vi "Up_SN.vi"(0 "Image Src":T8, 5 "ROIIn":string, 11 "error in":errorcluster) -> (4 "Image Out":T8(plugin-control), 6 "QR Code Report":T1={"Found?"=FALSE, "Data"="", "Bounding Box"=[], "Errors Corrected"=0, "Dimensions (Rows/Cols)"=0, "Version"=0, "QR Model"=0, "Stream Mode"=0, "Barcode Polarity"=-2, "Mirrored?"=FALSE, "Append Stream Position"=0, "Size of Append Stream"=0, "First EAN-128 ID"=0, "First Alternate Language ID"=0, "Append Stream ID"=0, "Minimum Edge Strength"=30, "Demodulation Mode"=-2, "Cell Sample Size"=-2, "Cell Filter Mode"=-2} {"Append Stream ID" format="%x"; "Cell Filter Mode" items=["Auto-detect"=-2, "Average"=0, "Median"=1, "Central Average"=2, "High Average"=3, "Low Average"=4, "Very High Average"=5, "Very Low Average"=6, "All Filters"=8]; "Cell Sample Size" items=["Auto-detect"=-2, "1x1"=1, "2x2"=2, "3x3"=3, "4x4"=4, "5x5"=5, "6x6"=6, "7x7"=7]; "Demodulation Mode" items=["Auto-detect"=-2, "Histogram"=0, "Local Contrast"=1, "Combination"=2, "All"=3]; "Barcode Polarity" items=["Auto-detect"=-2, "Black on White"=0, "White on Black"=1]; "Stream Mode" items=["Numeric", "AlphaNumeric", "Raw Bytes", "UCC/EAN-128 - In Tokens", "UCC/EAN-128 - In Data", "Extended Character Interpretation", "Kanji"]; "QR Model" items=["Auto-detect", "Micro", "Model 1", "Model 2"]; "Version" max=40 step=1}, 15 "error out":errorcluster)   [LabVIEW 2019]
uses:
  <vilib>/vision/Image Controls.llb/IMAQ Image.ctl
  <vilib>/vision/Instrument.llb/QR Code Report.ctl
  <vilib>/vision/Instrument.llb/QR Code Model Type.ctl
  <vilib>/vision/Instrument.llb/QR Code Stream Mode Type.ctl
  <vilib>/vision/Instrument.llb/Data Matrix Polarity.ctl
  <vilib>/vision/Instrument.llb/Demodulation Mode.ctl
  <vilib>/vision/Instrument.llb/Cell Sample Size.ctl
  <vilib>/vision/Instrument.llb/Cell Filter Mode.ctl
  <vilib>/vision/NI_Vision_Development_Module.lvlib
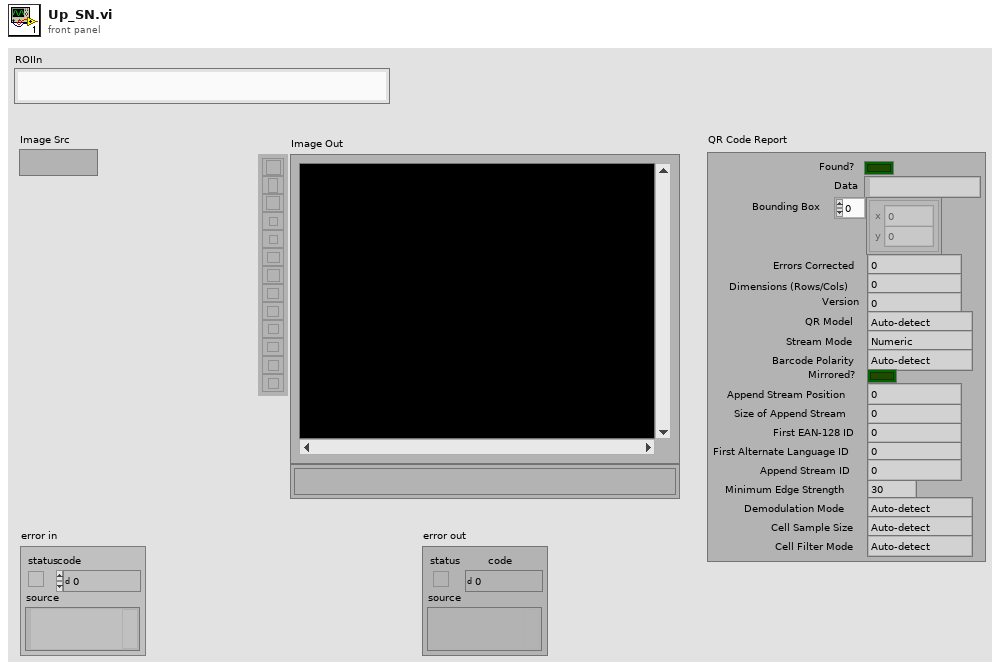
[diagram p1: front panel]
types:
  T1 = typedef "QR Code Report.ctl" = cluster{"Found?":bool, "Data":string, "Bounding Box":cluster{"x":sgl, "y":sgl}[], "Errors Corrected":u32, "Dimensions (Rows/Cols)":u32, "Version":u32, "QR Model":T2, "Stream Mode":T3, "Barcode Polarity":T4, "Mirrored?":bool, "Append Stream Position":u32, "Size of Append Stream":u32, "First EAN-128 ID":i32, "First Alternate Language ID":i32, "Append Stream ID":u32, "Minimum Edge Strength":u32, "Demodulation Mode":T5, "Cell Sample Size":T6, "Cell Filter Mode":T7}
  T2 = typedef "QR Code Model Type.ctl" = i32
  T3 = typedef "QR Code Stream Mode Type.ctl" = i32
  T4 = typedef "Data Matrix Polarity.ctl" = i32
  T5 = typedef "Demodulation Mode.ctl" = i32
  T6 = typedef "Cell Sample Size.ctl" = i32
  T7 = typedef "Cell Filter Mode.ctl" = i32
  T8 = typedef "IMAQ Image.ctl" = refnum<image>
  T9 = cluster{"Rotation Mode":enum32{"Unlimited", "0 Degrees", "90 Degrees", "180 Degrees", "270 Degrees"}, "Skip Location?":bool, "Edge Threshold":u32, "Demodulation Mode":i32, "Cell Sample Size":i32, "Cell Filter Mode":i32, "Skew Degrees Allowed":u32}[]
  T10 = typedef "Image Type" = u32
  T11 = typedef "IMAQ Rectangle" = cluster{"Left":i32, "Top":i32, "Right":i32, "Bottom":i32, "Rotation":dbl}
  T12 = cluster{"Matrix Dimensions (cells)":i32, "Barcode Polarity":i32, "Mirror Mode":i32, "QR Model":i32}
  T13 = cluster{"Rotation Mode":enum32{"Unlimited", "0 Degrees", "90 Degrees", "180 Degrees", "270 Degrees"}, "Skip Location?":bool, "Edge Threshold":u32, "Demodulation Mode":i32, "Cell Sample Size":i32, "Cell Filter Mode":i32, "Skew Degrees Allowed":u32}
  T14 = typedef "ROI Descriptor" = cluster{"Global Rectangle":i32[], "Contours":cluster{"ID":enum32{"External", "Internal"}, "Type":u32, "Coordinates":i32[]}[]}
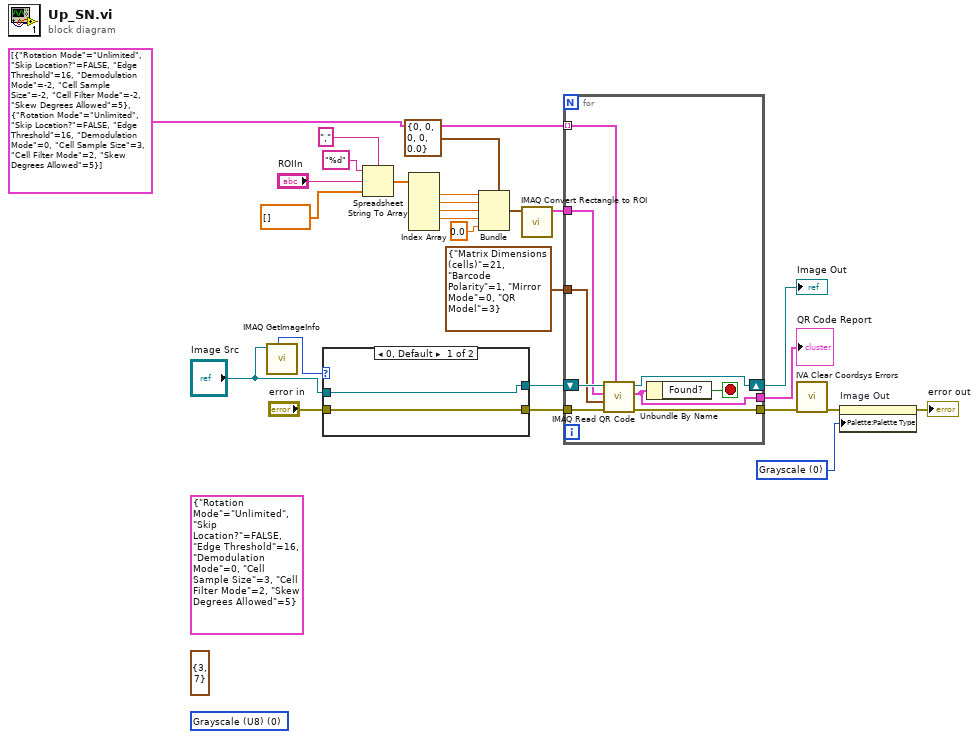
[diagram p0: block diagram]
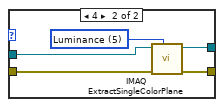
[diagram p2: hidden frame]
diagram:
  (unwired) T10 0 items=["Grayscale (U8)", "Grayscale (I16)", "Grayscale (SGL)", "Complex (CSG)", "RGB (U32)", "HSL (U32)", "RGB (U64)", "Grayscale (U16)"] ("Image Type")
  w19 = u32 0 items=["Grayscale", "Binary", "Gradient", "Rainbow", "Temperature", "User Defined", "Binary 16 Bit", "Gradient 16 Bit", "Rainbow 16 Bit", "Temperature 16 Bit", "User Defined 16 Bit"] ("Palette Type")
  (unwired) cluster{"Minimum Size":u32, "Maximum Size":u32} {"Minimum Size"=3, "Maximum Size"=7} ("QR Code Cell Size (pixels)")
  (unwired) T13 {"Rotation Mode"=enum."Unlimited", "Skip Location?"=FALSE, "Edge Threshold"=16, "Demodulation Mode"=0, "Cell Sample Size"=3, "Cell Filter Mode"=2, "Skew Degrees Allowed"=5} ("QR Search Options")
  n1 = call "IMAQ GetImageInfo"("Image"="Image Src") -> ("Image Type"=w3:T10)  [unwired: 3 in, 7 out]
  n2 = case shown="0, Default" w3 {
    tunnel: [w27 w32] -> w26
    tunnel: [w28 w31] -> w25
    tunnel: "error in" -> [w27 w30]
    tunnel: "Image Src" -> [w28 w29]
    frame 0, Default {
    }
    frame 4 {
      w33 = 5 items=["Red", "Green", "Blue", "Hue", "Saturation", "Luminance", "Value", "Intensity"] ("Color Plane")
      n3 = call "IMAQ ExtractSingleColorPlane"("Color Plane"=w33, "error in (no error)"=w30, "Image Src"=w29) -> ("error out"=w32:errorcluster, "Image Dst Out"=w31:T8)  [unwired: 1 in, 6 out]
    }
  }
  n4 = Spreadsheet String To Array(delimiter (Tab)=",", format string="%d", spreadsheet string="ROIIn", array type (2D Dbl)=dbl[] []) -> (array=w11:dbl[])
  n5 = Index Array(array=w11) -> (element #1=w10:dbl, element #2=w9:dbl, element #3=w8:dbl, element #4=w7:dbl)  [unwired: 5 in, 1 out]
  n6 = Bundle(cluster=T11 {"Left"=0, "Top"=0, "Right"=0, "Bottom"=0, "Rotation"=0.0} ("Rectangle"), "Left"=w10, "Top"=w9, "Right"=w8, "Bottom"=w7, "Rotation"=0.0) -> (w12:T11)
  n7 = call "IMAQ Convert Rectangle to ROI"("Rectangle"=w12) -> ("ROI Descriptor"=w5:T14)  [unwired: 8 in, 1 out]
  n8 = for {
    tunnel: T12 {"Matrix Dimensions (cells)"=21, "Barcode Polarity"=1, "Mirror Mode"=0, "QR Model"=3} ("QR Description Options") -> [w40]
    tunnel: w5 -> [w37]
    tunnel: T9 [{"Rotation Mode"=enum."Unlimited", "Skip Location?"=FALSE, "Edge Threshold"=16, "Demodulation Mode"=-2, "Cell Sample Size"=-2, "Cell Filter Mode"=-2, "Skew Degrees Allowed"=5}, {"Rotation Mode"=enum."Unlimited", "Skip Location?"=FALSE, "Edge Threshold"=16, "Demodulation Mode"=0, "Cell Sample Size"=3, "Cell Filter Mode"=2, "Skew Degrees Allowed"=5}] ("Array") -> [w36] mode=indexing
    tunnel: [w35] -> w2
    shift-right: [w38] -> w20
    shift-left: w25 -> [w41]
    tunnel: w26 -> [w42]
    tunnel: [w39] -> w23
    stop <- w34 stop-if-true
    n9 = call "IMAQ Read QR Code"("QR Search Options"=w36, "error in (no error)"=w42, "QR Description Options"=w40, "ROI Descriptor"=w37, "Image"=w41) -> ("error out"=w39:errorcluster, "QR Code Report"=w35:T1, "Image (duplicate)"=w38:T8)  [unwired: 2 in, 2 out]
    n10 = Unbundle By Name(w35) -> ("Found?"=w34:bool)
  }
  "Image Out" <- w20
  "QR Code Report" <- w2
  n11 = call <vilib>:"IVA Clear Coordsys Errors.vi"("error in (no error)"=w23) -> ("error out"=w22:errorcluster)  [unwired: 10 in]
  n12 = property on="Image Out" class="ImageControl"(error in=w22, "Palette:Palette Type"=w19) -> (error out=→"error out":errorcluster)  [unwired: 1 in, 1 out]
